vi "Read Strg.vi"(8 "error in (no error)":errorcluster, 11 "ClassData in":refnum<class "ClassData.lvclass">) -> (0 "error out":errorcluster, 2 "Strg":string, 3 "ClassData out":refnum<class "ClassData.lvclass">)   [LabVIEW 2018, in "ClassData.lvclass"]
uses:
  ClassData.lvclass
  ClassData.lvclass/ClassData.ctl
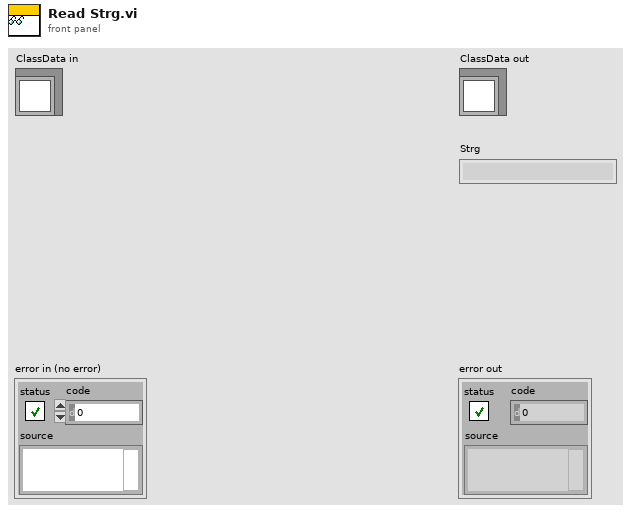
[diagram p1: front panel]
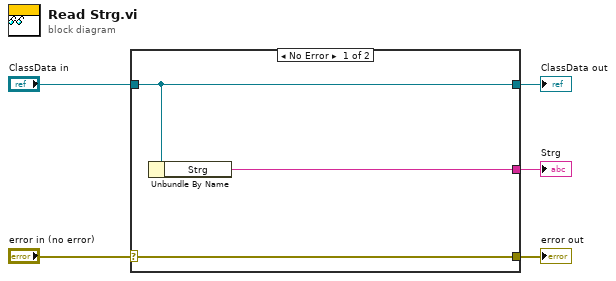
[diagram p0: block diagram]
diagram:
  n1 = case shown="No Error" "error in (no error)" {
    selector: "error in (no error)" -> [w8 w9]
    tunnel: [w8 w9] -> w4
    tunnel: [w7 w10] -> w2
    tunnel: "ClassData in" -> [w7 w10]
    tunnel: [w6 _] -> w1
    frame No Error {
      n2 = Unbundle By Name(w7) -> ("Strg"=w6:string)
    }
    frame Error {
    }
  }
  "error out" <- w4
  "ClassData out" <- w2
  "Strg" <- w1
